vi "Speed Test Single VI.vi"() -> ()   [LabVIEW 2016, in "Data.ITX.lvclass"]
uses:
  Data.ITX/Data.ITX.lvclass
panel:
  in  "Numeric 2":i32
  in  "Numeric":i32
  out "elapsed time (s)":dbl format="%#_6p"
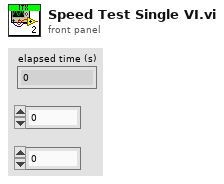
[diagram p1: front panel]
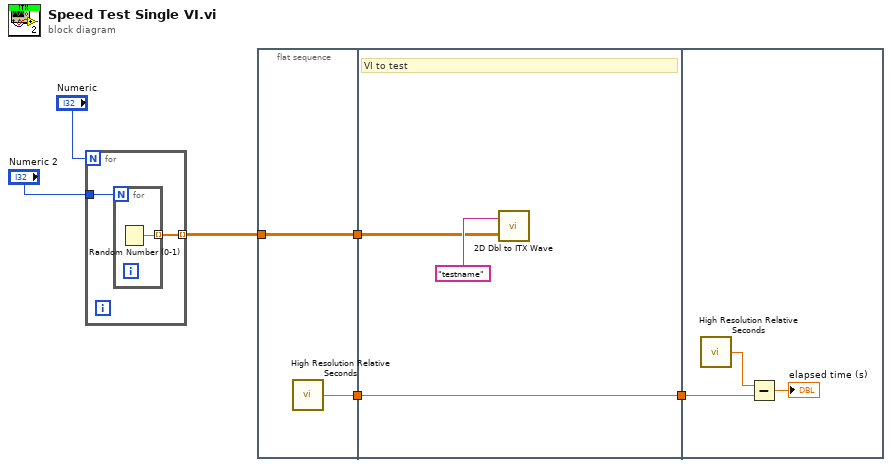
[diagram p0: block diagram]
diagram:
  n1 = for {
    N: "Numeric" -> [_]
    tunnel: [w8] -> w3 mode=indexing
    tunnel: "Numeric 2" -> [w7]
    n2 = for {
      N: w7 -> [_]
      tunnel: [w9] -> w8 mode=indexing
      n3 = Random Number (0-1)() -> (number: 0 to 1=w9:dbl)
    }
  }
  n4 = flat-sequence {
    tunnel: [w11] -> w6
    tunnel: [w10] -> w5
    tunnel: w3 -> [w10]
    tunnel: w6 -> [w14]
    tunnel: [w14] -> w4
    tunnel: w5 -> [w12]
    tunnel: w4 -> [w16]
    frame #0 {
      n5 = call <vilib>:"High Resolution Relative Seconds.vi"() -> ("relative seconds"=w11:dbl)
    }
    frame #1 {
      # "VI to test"
      n6 = call "2D Dbl to ITX Wave.vi"("2D Array"=w12, "Wavename"="testname") -> ()  [unwired: 1 out]
    }
    frame #2 {
      n7 = call <vilib>:"High Resolution Relative Seconds.vi"() -> ("relative seconds"=w17:dbl)
      n8 = Subtract(x=w17, y=w16) -> (x-y=→"elapsed time (s)":dbl)
    }
  }
